vi "高温告警对话框.vi"() -> (3 "T button?":bool)   [LabVIEW 2016]
panel:
  out "告警字符串":string
  in  "取消告警":bool
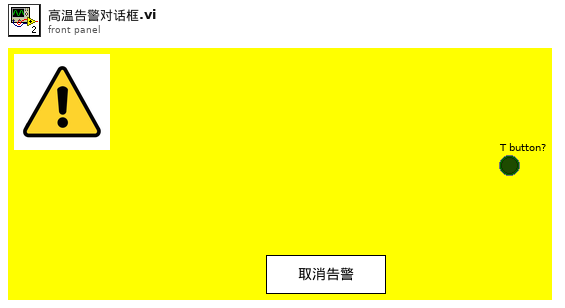
[diagram p1: front panel]
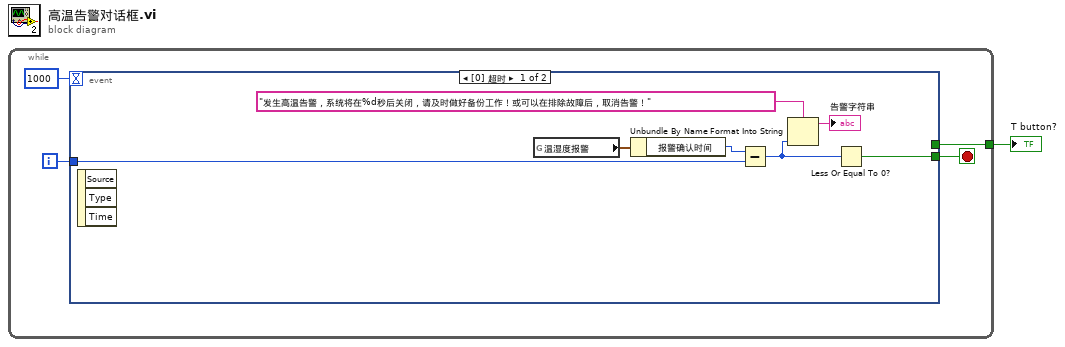
[diagram p0: block diagram]
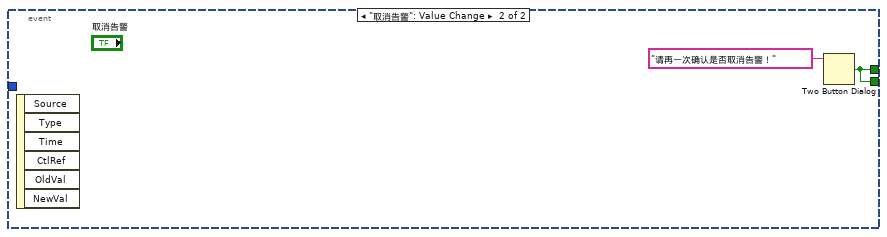
[diagram p2: hidden frame]
diagram:
  n1 = while {
    tunnel: [w5] -> w1
    i -> [w2]
    stop <- w4 stop-if-true
    n2 = event shown="[0] 超时" {
      selector: _ -> [_ _]
      dyn-events: _ -> [_ _]
      timeout: 1000 -> [_ _]
      tunnel: [_ w13] -> w5
      tunnel: [w8 w13] -> w4
      tunnel: w2 -> [w12 _]
      event Timeout {
        n3 = event-data() -> ()  [unwired: 1 in, 3 out]
        n4 = global read "系统设置全局变量.vi" "温湿度报警"() -> (w7:cluster{"温度报警":u16, "湿度报警":u16, "报警确认时间":u16})
        n5 = Unbundle By Name(w7) -> ("报警确认时间"=w6:u16)
        n6 = Subtract(x=w6, y=w12) -> (x-y=w9:i32)
        n7 = Format Into String(format string="发生高温告警，系统将在%d秒后关闭，请及时做好备份工作！或可以在排除故障后，取消告警！" ("格式字符串"), w9) -> (resulting string=→"告警字符串":string)  [unwired: 2 in, 1 out]
        n8 = Less Or Equal To 0?(x=w9) -> (x <= 0?=w8:bool)
      }
      event "取消告警": Value Change {
        n9 = event-data() -> ()  [unwired: 1 in, 6 out]
        n10 = Two Button Dialog(message="请再一次确认是否取消告警！" ("消息")) -> (T button?=w13:bool)  [unwired: 2 in]
      }
    }
  }
  "T button?" <- w1
